vi "BuildServer Globals.vi"() -> ()   [LabVIEW 2017]
panel:
  in  "BuildWorker Dir":path
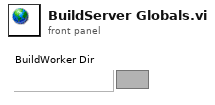
[diagram p1: front panel]
diagram:
